vi "Write Instrument Model.vi"(8 "error in (no error)":errorcluster, 10 "Instrument Model":string, 11 "SG Path in":refnum<class "SG Path.lvclass">) -> (0 "error out":errorcluster, 3 "SG Path out":refnum<class "SG Path.lvclass">)   [LabVIEW 2023, in "RFFixtureCharact.Public.lvlib" / "SG Path.lvclass"]
uses:
  SG Path.lvclass
  SG Path.lvclass/SG Path.ctl
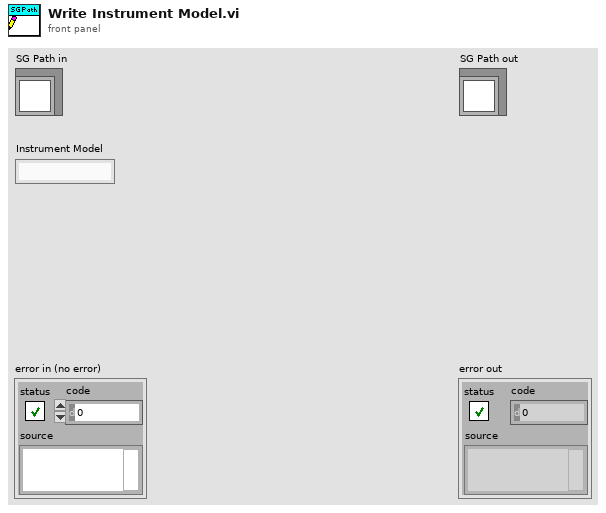
[diagram p1: front panel]
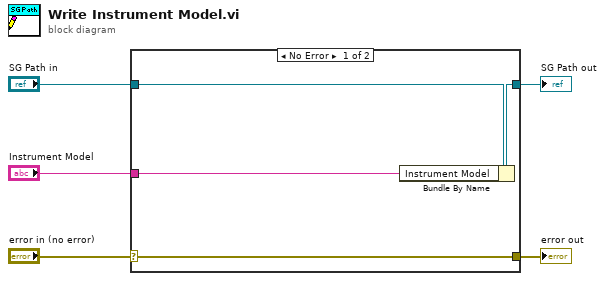
[diagram p0: block diagram]
diagram:
  n1 = case shown="No Error" "error in (no error)" {
    selector: "error in (no error)" -> [w9 w10]
    tunnel: [w9 w10] -> w4
    tunnel: [w7 w11] -> w2
    tunnel: "SG Path in" -> [w8 w11]
    tunnel: "Instrument Model" -> [w6 _]
    frame No Error {
      n2 = Bundle By Name(cluster=w8, "Instrument Model"=w6) -> (w7:refnum<class "SG Path.lvclass">)
    }
    frame Error {
    }
  }
  "error out" <- w4
  "SG Path out" <- w2
